vi "Archery_About.vi"() -> ()   [LabVIEW 2014]
panel:
  in  "OK Button":bool
  # "Archery Simulator v1.0\nCopyright © 2021 David Hsu"
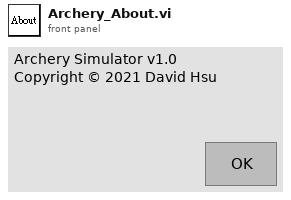
[diagram p1: front panel]
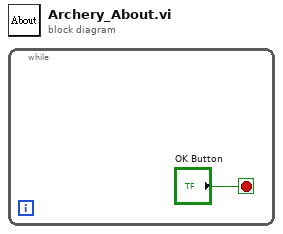
[diagram p0: block diagram]
diagram:
  n1 = while {
    stop <- "OK Button" stop-if-true
  }
